vi "Binary_To_Decimal.vi"() -> ()   [LabVIEW 2020]
panel:
  in  "Bit 1 (LSB)":bool
  in  "Bit 2":bool
  in  "Bit 3":bool
  in  "Bit 4 (MSB)":bool
  out "Digital Output":dbl
  # "Binary to Decimal"
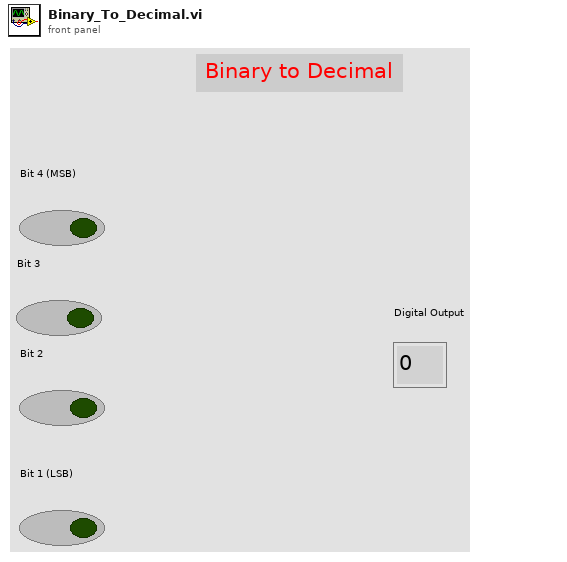
[diagram p1: front panel]
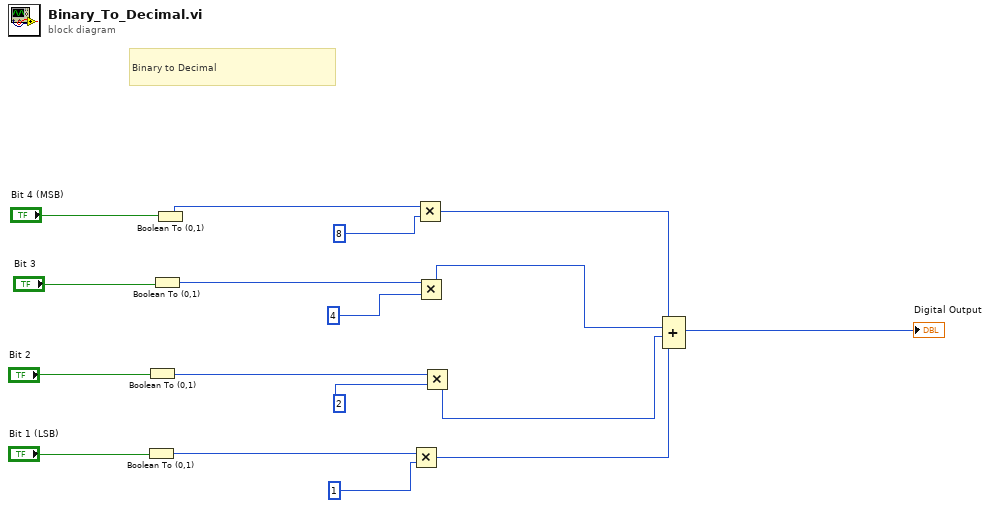
[diagram p0: block diagram]
diagram:
  # "Binary to Decimal"
  n1 = Boolean To (0,1)(Boolean="Bit 1 (LSB)") -> (0, 1=w6:i16)
  n2 = Boolean To (0,1)(Boolean="Bit 2") -> (0, 1=w7:i16)
  n3 = Boolean To (0,1)(Boolean="Bit 3") -> (0, 1=w8:i16)
  n4 = Boolean To (0,1)(Boolean="Bit 4 (MSB)") -> (0, 1=w13:i16)
  n5 = Multiply(x=w6, y=1) -> (x*y=w2:i32)
  n6 = Multiply(x=w13, y=8) -> (x*y=w5:i32)
  n7 = Multiply(x=w8, y=4) -> (x*y=w4:i32)
  n8 = Multiply(x=w7, y=2) -> (x*y=w3:i32)
  n9 = Compound Arithmetic op=ADD(w5, w4, w3, w2) -> (→"Digital Output":i32)
